vi "query 2.vi"() -> (27 "error out 2":errorcluster)   [LabVIEW 2019]
uses:
  <vilib>/Utility/NIReport.llb/Report Type.ctl
  <vilib>/addons/database/Connection.llb/DB Tools Open Connec (String).vi
  <vilib>/addons/_office/excel.llb/Excel Easy Table (str).vi
  <vilib>/addons/database/_DB Variant To Data/Database Variant To Data.xnode
  <vilib>/Utility/NIReport.llb/NI_report.lvclass
  <vilib>/addons/database/NI_Database_API.lvlib
  <vilib>/Utility/NIReport.llb/NI_ReportGenerationCore.lvlib
  <vilib>/addons/_office/NI_ReportGenerationToolkit.lvlib
  database.lvlib
panel:
  out "Table":string[][](table)
  in  "error in (no error)":errorcluster
  in  "pallet_sit sel":bool
  in  "swl sel":bool
  in  "SWR sel":bool
  in  "curv_sit sel":bool
  in  "def_type sel":bool
  in  "GB_sit sel":bool
  in  "UNTIL":timestamp
  in  "FROM":timestamp
  in  "pallet_num sel":bool
  in  "time select":bool
  in  "pallet number":i16
  in  "Pallet-sit":u16(ring) items=["normal", "warning", "error"]
  in  "CURV_SITUATION":u16(ring) items=["normal", "error"]
  in  "SWR":u16(ring) items=["normal", "error"]
  in  "SWL":u16(ring) items=["normal", "error"]
  in  "GB_SITUATION":u16(ring) items=["normal", "warning", "error"]
  in  "DEFECTS_TYPE":u16(ring) items=["gap", "hole"]
  in  "TIME":u16(ring) items=["selected period", "last day", "last week", "last mounth", "Last Turn"]
  in  "Close Square":bool
  in  "Search Button 2":bool
  in  "Save As Button 2":bool
  in  "Base Path":path=path "C:/excel files"
  # "DPIS"
  # "REPORT"
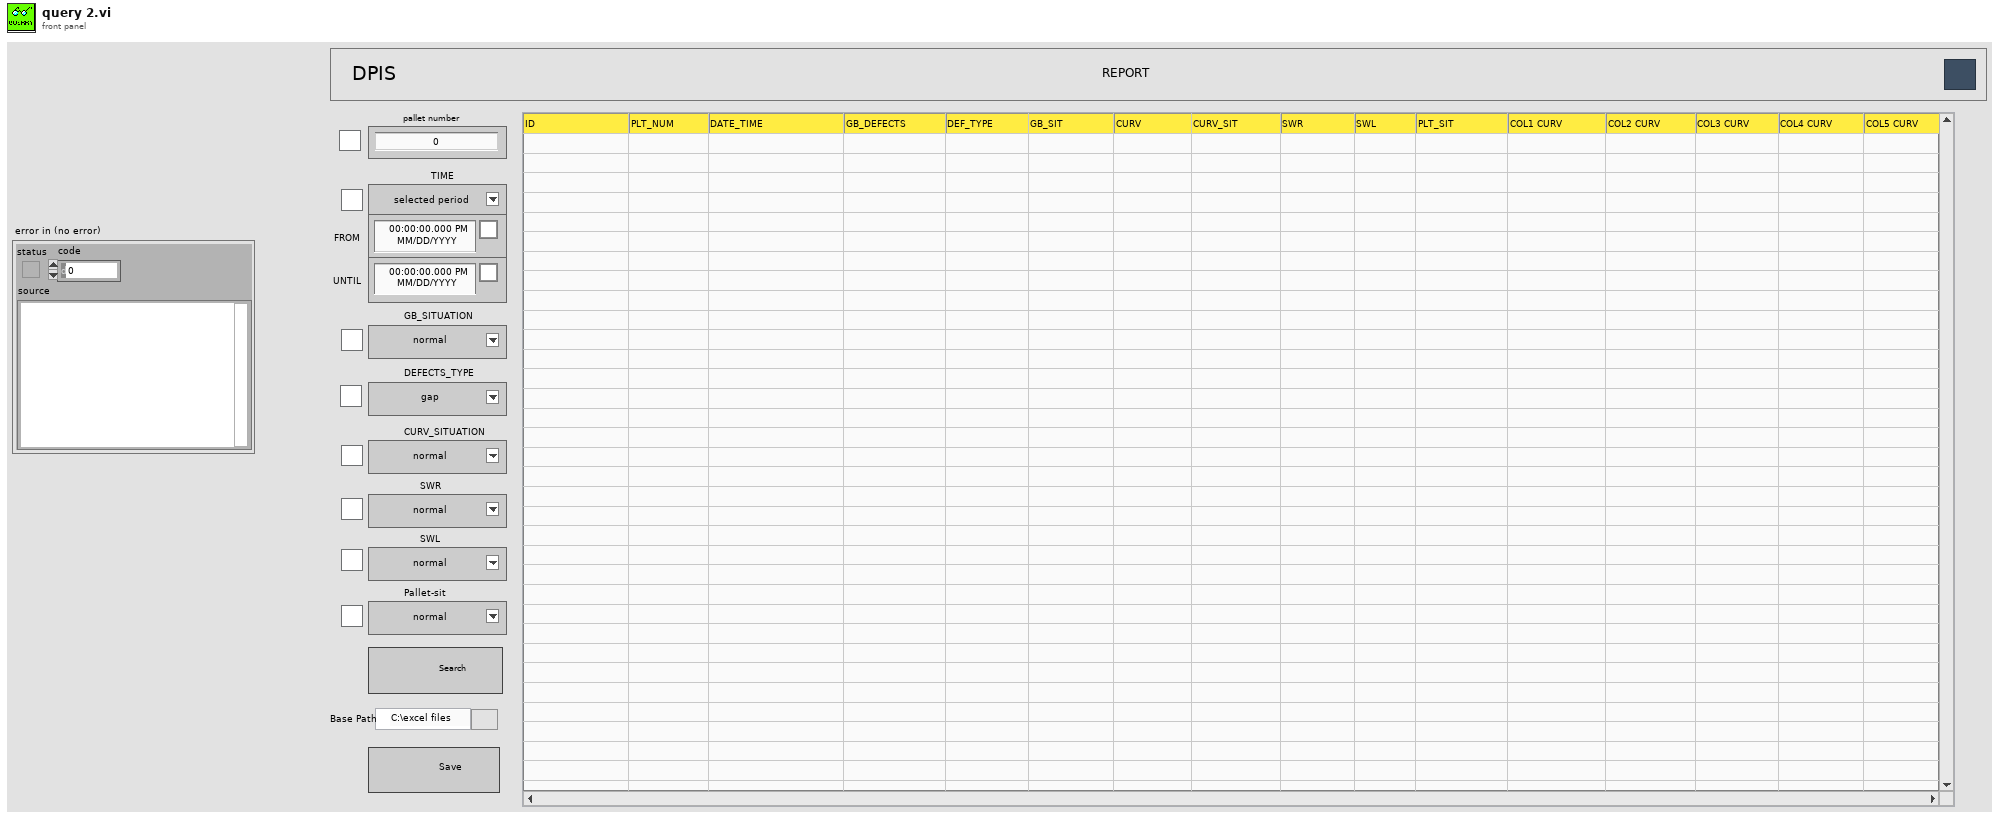
[diagram p1: front panel]
types:
  T1 = enum16{"maximized", "minimized", "normal", "no change"}
  T2 = typedef "NI_ReportGenerationCore.lvlib/Report Type.ctl" = enum16{"HTML", "Word", "Excel"}
  T3 = typedef "NI_Database_API.lvlib/Conn ObjectReference.ctl" = refnum<k1>
  T4 = cluster{"plt number dis":i16, "Table Name":string, "Database Name":string, "DB days to save":i16, "IP #":string, "Img Path":path, "Port":u16, "time out":u16, "madule path":path, "IP # speed":string, "counting device":enum16{"Sensors", "Line Speed", "Sensors&Speed"}}
  T5 = typedef "LVDateTimeRec.ctl" = cluster{"fractional second":dbl, "second":i32, "minute":i32, "hour":i32, "day of month":i32, "month":i32, "year":i32, "day of week":i32, "day of year":i32, "DST":i32}
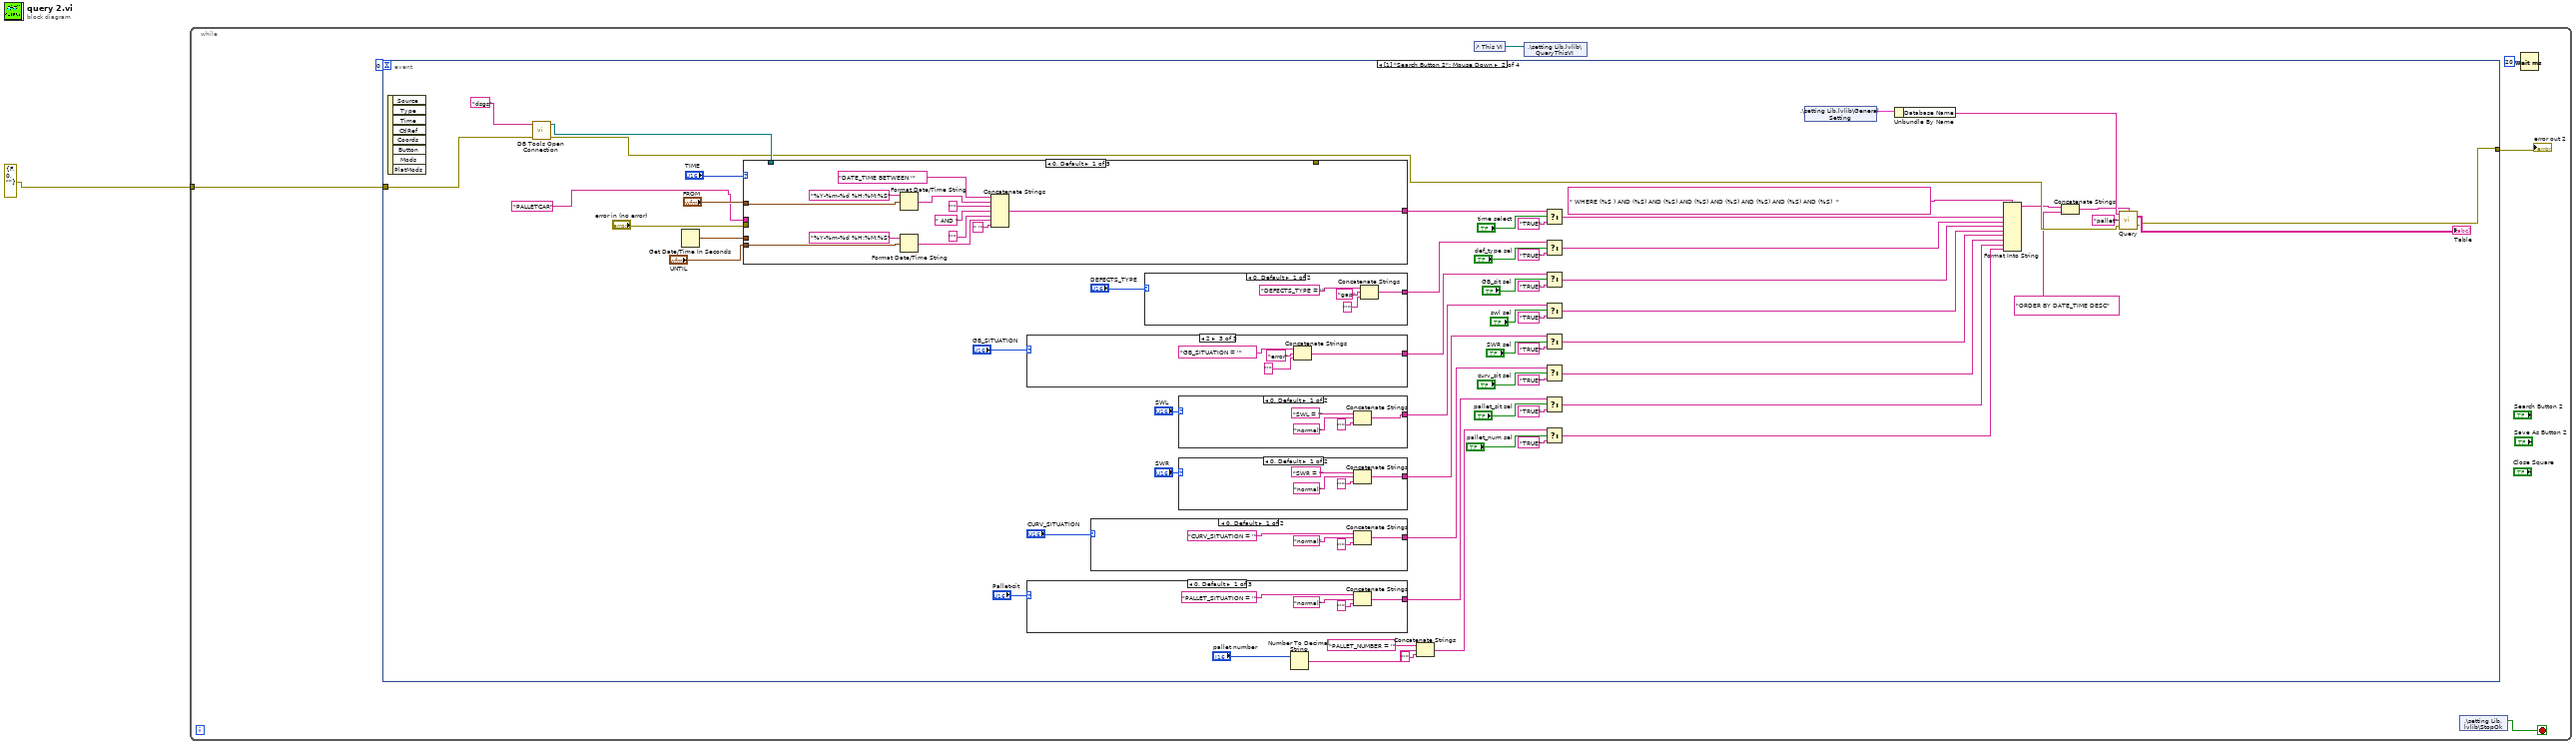
[diagram p0: block diagram]
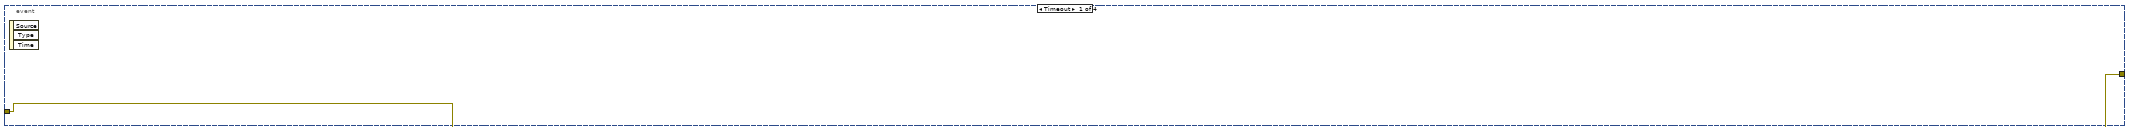
[diagram p2: hidden frame]
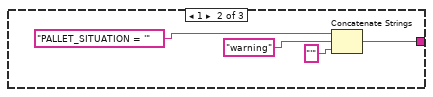
[diagram p3: hidden frame]
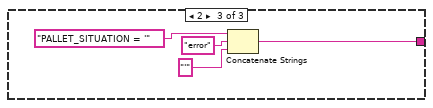
[diagram p4: hidden frame]
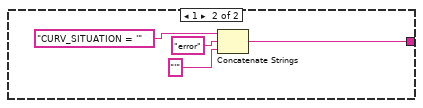
[diagram p5: hidden frame]
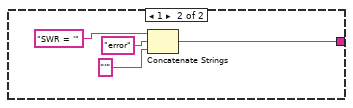
[diagram p6: hidden frame]
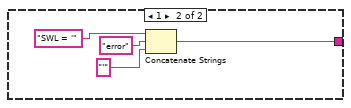
[diagram p7: hidden frame]
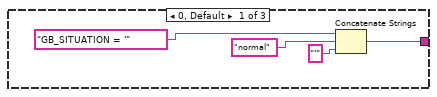
[diagram p8: hidden frame]
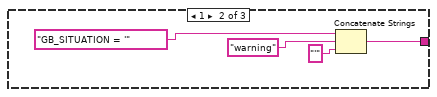
[diagram p9: hidden frame]
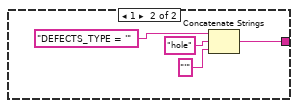
[diagram p10: hidden frame]
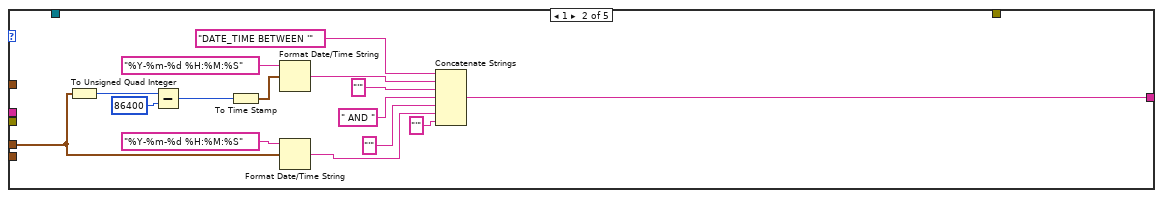
[diagram p11: hidden frame]
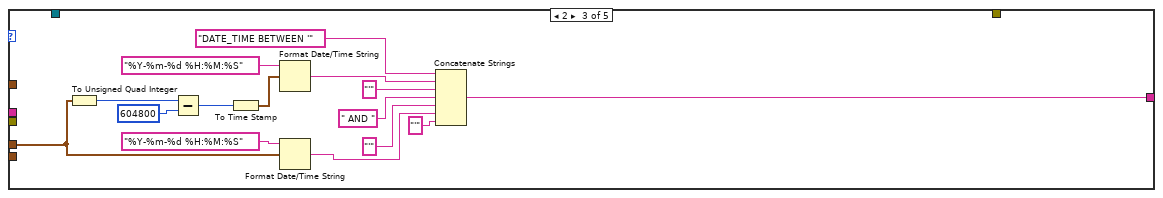
[diagram p12: hidden frame]
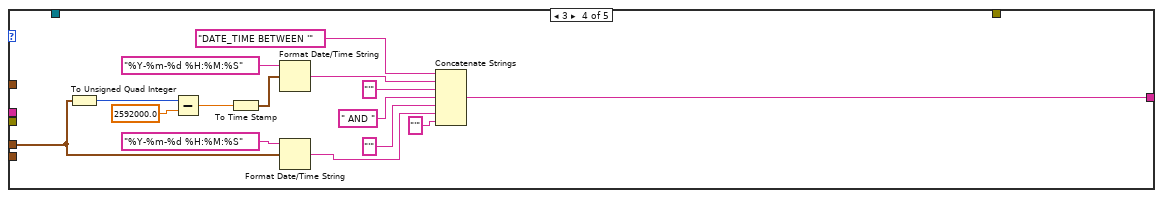
[diagram p13: hidden frame]
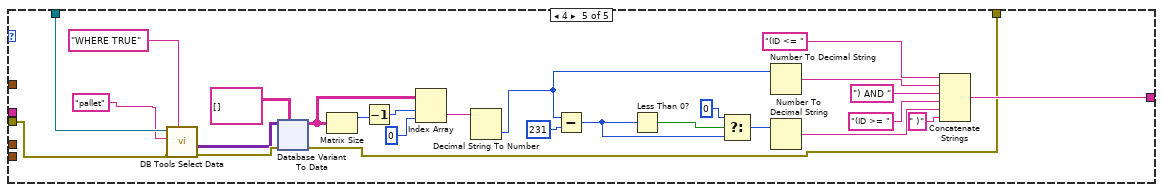
[diagram p14: hidden frame]
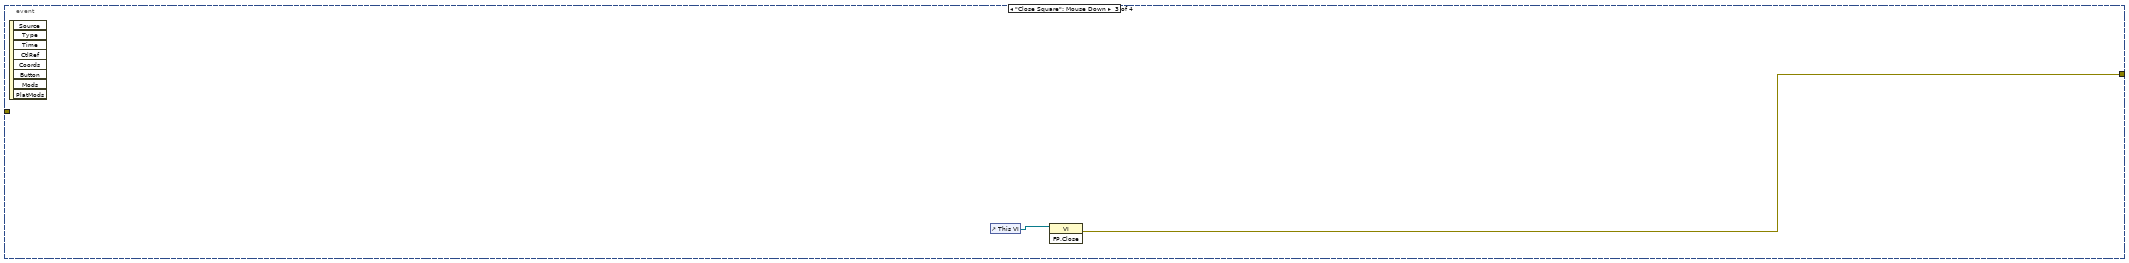
[diagram p15: hidden frame]
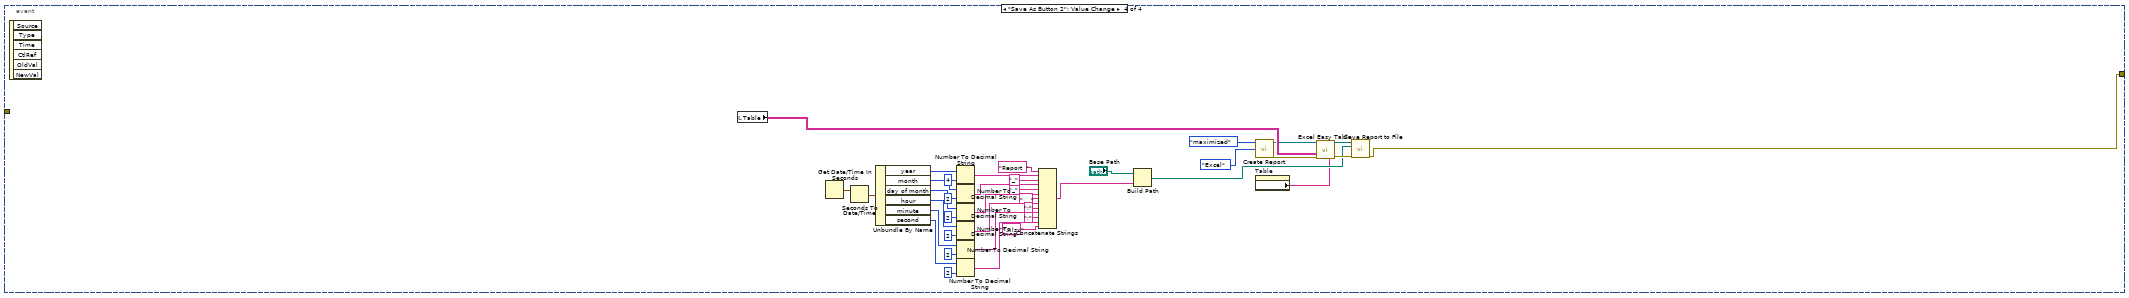
[diagram p16: hidden frame]
diagram:
  n1 = while {
    tunnel: errorcluster {"status"=FALSE, "code"=0, "source"=""} ("error in (no error)") -> [w2]
    stop <- w3 stop-if-true
    n2 = event shown="[1] \"Search Button 2\": Mouse Down" {
      selector: _ -> [_ _ _ _]
      dyn-events: _ -> [_ _ _ _]
      timeout: 0 -> [_ _ _ _]
      tunnel: [w8 w12 w253 w255] -> w4
      tunnel: w2 -> [w8 w18 _ _]
      event Timeout {
        n3 = event-data() -> ()  [unwired: 1 in, 3 out]
      }
      event "Search Button 2": Mouse Down {
        n4 = event-data() -> ()  [unwired: 1 in, 8 out]
        n5 = call-poly <vilib>:"DB Tools Open Connection.vi"("error in (no error)"=w18, "connection information"="dsgs" ("database name")) -> ("error out"=w13:errorcluster, "connection reference"=w19:T3)  [unwired: 6 in]
        n6 = Get Date/Time In Seconds() -> (seconds since 1Jan1904=w62:timestamp)
        n7 = case shown="0, Default" "TIME" {
          tunnel: "FROM" -> [w134 _ _ _ _]
          tunnel: "UNTIL" -> [w132 _ _ _ _]
          tunnel: [w127 w142 w153 w168 w193] -> w35
          tunnel: w62 -> [_ w140 w155 w170 _]
          tunnel: "error in (no error)" -> [_ _ _ _ w185]
          tunnel: [_ _ _ _ w186] -> _
          tunnel: "PALLETCAR" ("database name") -> [_ _ _ _ _]
          tunnel: w19 -> [_ _ _ _ w184]
          frame 0, Default {
            n8 = Format Date/Time String(time format string (%c)="%Y-%m-%d %H:%M:%S", seconds (now)=w134) -> (date/time string=w133:string)  [unwired: 1 in]
            n9 = Format Date/Time String(time format string (%c)="%Y-%m-%d %H:%M:%S", seconds (now)=w132) -> (date/time string=w129:string)  [unwired: 1 in]
            n10 = Concatenate Strings("DATE_TIME BETWEEN '" ("condition"), w133, "'" ("string"), " AND " ("time format string (%c)"), "'" ("string"), w129, " '" ("string")) -> (w127:string)
          }
          frame 1 {
            n11 = To Unsigned Quad Integer(1:w140) -> (0:w150:u64)
            n12 = Subtract(x=w150, y=u64 86400) -> (x-y=w152:u64)
            n13 = To Time Stamp(1:w152) -> (0:w141:timestamp)
            n14 = Format Date/Time String(time format string (%c)="%Y-%m-%d %H:%M:%S", seconds (now)=w141) -> (date/time string=w146:string)  [unwired: 1 in]
            n15 = Format Date/Time String(time format string (%c)="%Y-%m-%d %H:%M:%S", seconds (now)=w140) -> (date/time string=w143:string)  [unwired: 1 in]
            n16 = Concatenate Strings("DATE_TIME BETWEEN '" ("condition"), w146, "'" ("string"), " AND " ("time format string (%c)"), "'" ("string"), w143, "'" ("string")) -> (w142:string)
          }
          frame 2 {
            n17 = To Unsigned Quad Integer(1:w155) -> (0:w158:u64)
            n18 = Subtract(x=w158, y=u64 604800) -> (x-y=w156:u64)
            n19 = To Time Stamp(1:w156) -> (0:w154:timestamp)
            n20 = Format Date/Time String(time format string (%c)="%Y-%m-%d %H:%M:%S", seconds (now)=w154) -> (date/time string=w163:string)  [unwired: 1 in]
            n21 = Format Date/Time String(time format string (%c)="%Y-%m-%d %H:%M:%S", seconds (now)=w155) -> (date/time string=w160:string)  [unwired: 1 in]
            n22 = Concatenate Strings("DATE_TIME BETWEEN '" ("condition"), w163, "'" ("condition"), " AND " ("time format string (%c)"), "'" ("string"), w160, "'" ("string")) -> (w153:string)
          }
          frame 3 {
            n23 = To Unsigned Quad Integer(1:w170) -> (0:w172:u64)
            n24 = Subtract(x=w172, y=2592000.0) -> (x-y=w173:dbl)
            n25 = To Time Stamp(1:w173) -> (0:w169:timestamp)
            n26 = Format Date/Time String(time format string (%c)="%Y-%m-%d %H:%M:%S", seconds (now)=w169) -> (date/time string=w178:string)  [unwired: 1 in]
            n27 = Format Date/Time String(time format string (%c)="%Y-%m-%d %H:%M:%S", seconds (now)=w170) -> (date/time string=w181:string)  [unwired: 1 in]
            n28 = Concatenate Strings("DATE_TIME BETWEEN '" ("condition"), w178, "'" ("condition"), " AND " ("time format string (%c)"), "'" ("string"), w181, "'" ("string")) -> (w168:string)
          }
          frame 4 {
            n29 = call <vilib>:"DB Tools Select Data.vi"("condition"="WHERE TRUE" ("format string"), "error in (no error)"=w185, "table"="pallet", "connection reference"=w184) -> ("error out"=w208:errorcluster, "data"=w207:variant[][])  [unwired: 2 in, 1 out]
            n30 = xnode "Database Variant To Data"("database variant"=w207, "error in (no error)"=w208, "type"=string[][] []) -> ("data"=w192:string[][], "error out"=w186:errorcluster)
            n31 = Matrix Size(0:w192) -> (1:w191:i32)  [unwired: 1 out]
            n32 = Decrement(x=w191) -> (x-1=w190:i32)
            n33 = Index Array(array=w192, index (row)=w190, index (col)=0 ("disabled index (col)")) -> (element=w188:string)
            n34 = Decimal String To Number(string=w188) -> (number=w187:i32)  [unwired: 2 in, 1 out]
            n35 = Subtract(x=w187, y=231) -> (x-y=w202:i32)
            n36 = Less Than 0?(x=w202) -> (x < 0?=w201:bool)
            n37 = Select(t=0 ("y"), s=w201, f=w202) -> (s? t:f=w203:i32)
            n38 = Number To Decimal String(number=w187) -> (decimal integer string=w200:string)  [unwired: 1 in]
            n39 = Number To Decimal String(number=w203) -> (decimal integer string=w204:string)  [unwired: 1 in]
            n40 = Concatenate Strings("(ID <= " ("condition"), w200, ") AND " ("string"), "(ID >= " ("string"), w204, " )" ("string")) -> (w193:string)
          }
        }
        n41 = case shown="2" "GB_SITUATION" {
          tunnel: [w106 w110 w114] -> w49
          frame 0, Default {
            n42 = Concatenate Strings("GB_SITUATION = '" ("string"), "normal" ("string"), "'" ("string")) -> (w106:string)
          }
          frame 1 {
            n43 = Concatenate Strings("GB_SITUATION = '" ("string"), "warning" ("string"), "'" ("string")) -> (w110:string)
          }
          frame 2 {
            n44 = Concatenate Strings("GB_SITUATION = '" ("string"), "error" ("string"), "'" ("string")) -> (w114:string)
          }
        }
        n45 = case shown="0, Default" "Pallet-sit" {
          tunnel: [w70 w74 w78] -> w41
          frame 0, Default {
            n46 = Concatenate Strings("PALLET_SITUATION = '" ("string"), "normal" ("string"), "'" ("string")) -> (w70:string)
          }
          frame 1 {
            n47 = Concatenate Strings("PALLET_SITUATION = '" ("string"), "warning" ("string"), "'" ("string")) -> (w74:string)
          }
          frame 2 {
            n48 = Concatenate Strings("PALLET_SITUATION = '" ("string"), "error" ("string"), "'" ("string")) -> (w78:string)
          }
        }
        n49 = case shown="0, Default" "CURV_SITUATION" {
          tunnel: [w82 w86] -> w43
          frame 0, Default {
            n50 = Concatenate Strings("CURV_SITUATION = '" ("string"), "normal" ("string"), "'" ("string")) -> (w82:string)
          }
          frame 1 {
            n51 = Concatenate Strings("CURV_SITUATION = '" ("string"), "error" ("string"), "'" ("string")) -> (w86:string)
          }
        }
        n52 = case shown="0, Default" "DEFECTS_TYPE" {
          tunnel: [w118 w122] -> w56
          frame 0, Default {
            n53 = Concatenate Strings("DEFECTS_TYPE = '" ("string"), "gap" ("string"), "'" ("string")) -> (w118:string)
          }
          frame 1 {
            n54 = Concatenate Strings("DEFECTS_TYPE = '" ("string"), "hole" ("string"), "'" ("string")) -> (w122:string)
          }
        }
        n55 = case shown="0, Default" "SWL" {
          tunnel: [w98 w102] -> w47
          frame 0, Default {
            n56 = Concatenate Strings("SWL = '" ("string"), "normal" ("string"), "'" ("string")) -> (w98:string)
          }
          frame 1 {
            n57 = Concatenate Strings("SWL = '" ("string"), "error" ("string"), "'" ("string")) -> (w102:string)
          }
        }
        n58 = case shown="0, Default" "SWR" {
          tunnel: [w90 w94] -> w45
          frame 0, Default {
            n59 = Concatenate Strings("SWR = '" ("string"), "normal" ("string"), "'" ("string")) -> (w90:string)
          }
          frame 1 {
            n60 = Concatenate Strings("SWR = '" ("string"), "error" ("string"), "'" ("string")) -> (w94:string)
          }
        }
        n61 = Number To Decimal String(number="pallet number") -> (decimal integer string=w61:string)  [unwired: 1 in]
        n62 = Concatenate Strings("PALLET_NUMBER = '" ("string"), w61, "'" ("string")) -> (w39:string)
        n63 = Select(t=w35, s="time select", f="TRUE") -> (s? t:f=w34:string)
        n64 = Select(t=w56, s="def_type sel", f="TRUE") -> (s? t:f=w33:string)
        n65 = Select(t=w49, s="GB_sit sel", f="TRUE") -> (s? t:f=w32:string)
        n66 = Select(t=w47, s="swl sel", f="TRUE") -> (s? t:f=w31:string)
        n67 = Select(t=w45, s="SWR sel", f="TRUE") -> (s? t:f=w30:string)
        n68 = Select(t=w43, s="curv_sit sel", f="TRUE") -> (s? t:f=w29:string)
        n69 = Select(t=w41, s="pallet_sit sel", f="TRUE") -> (s? t:f=w28:string)
        n70 = Select(t=w39, s="pallet_num sel", f="TRUE") -> (s? t:f=w27:string)
        n71 = shared-variable ".\\setting Lib.lvlib\\General Setting"() -> (w17:T4)  [unwired: 1 in, 1 out]
        n72 = Unbundle By Name(w17) -> ("Database Name"=w16:string)
        n73 = Format Into String(format string=" WHERE (%S ) AND (%S) AND (%S) AND (%S) AND (%S) AND (%S) AND (%S) AND (%S)  ", w34, w33, w32, w31, w30, w29, w28, w27) -> (resulting string=w11:string)  [unwired: 2 in, 1 out]
        n74 = Concatenate Strings(w11, "ORDER BY DATE_TIME DESC" ("string")) -> (w9:string)
        n75 = call "Query.vi"("Condition"=w9, "Error in"=w13, "Table Name"="pallet", "Connection Name"=w16) -> ("Error out"=w12:errorcluster, "data"=→"Table":string[][])
      }
      event "Close Square": Mouse Down {
        n76 = event-data() -> ()  [unwired: 1 in, 8 out]
        n77 = control-ref of="This VI"() -> (w254:refnum<vi>)
        n78 = invoke class="VI" method="FP.Close"(reference=w254) -> (error out=w253:errorcluster)  [unwired: 2 in, 2 out]
      }
      event "Save As Button 2": Value Change {
        n79 = event-data() -> ()  [unwired: 1 in, 6 out]
        n80 = local read "Table"() -> (w293:string[][])
        n81 = Get Date/Time In Seconds() -> (seconds since 1Jan1904=w290:timestamp)
        n82 = Seconds To Date/Time(time stamp (now)=w290) -> (date time rec=w289:T5)  [unwired: 1 in]
        n83 = Unbundle By Name(w289) -> ("year"=w288:i32, "month"=w287:i32, "day of month"=w286:i32, "hour"=w285:i32, "minute"=w284:i32, "second"=w283:i32)
        n84 = Number To Decimal String(number=w288, width (-)=i16 4) -> (decimal integer string=w282:string)
        n85 = Number To Decimal String(number=w287, width (-)=i16 2) -> (decimal integer string=w280:string)
        n86 = Number To Decimal String(number=w286, width (-)=i16 2) -> (decimal integer string=w278:string)
        n87 = Number To Decimal String(number=w285, width (-)=i16 2) -> (decimal integer string=w276:string)
        n88 = Number To Decimal String(number=w284, width (-)=i16 2) -> (decimal integer string=w274:string)
        n89 = Number To Decimal String(number=w283, width (-)=i16 2) -> (decimal integer string=w272:string)
        n90 = Concatenate Strings("Report  " ("string"), w282, "_" ("string"), w280, "_" ("string"), w278, "    " ("string"), w276, ";" ("string"), w274, ";" ("string"), w272, ".xlsx" ("string")) -> (w270:string)
        n91 = Build Path(base path="Base Path", name or relative path=w270) -> (appended path=w260:path)
        n92 = property on="Table" class="Tbl (strict)"() -> ("Column Headers[]"=w257:string[])  [unwired: 2 in, 2 out]
        n93 = call <vilib>:"Create Report.vi"("window state (normal)"=T1."maximized", "report type"=Report_Type."Excel") -> ("report out"=w259:refnum<class "NI_report.lvclass">, "error out"=w258:errorcluster)  [unwired: 12 in]
        n94 = call-poly <vilib>:"Excel Easy Table.vi"("report in"=w259, "text data"=w293, "error in (no error)"=w258, "column headers"=w257) -> ("report out"=w261:refnum<class "NI_report.lvclass">, "error out"=w262:errorcluster)  [unwired: 7 in, 3 out]
        n95 = call-dynamic "Save Report to File.vi"("report in"=w261, "report file path"=w260, "error in (no error)"=w262) -> ("error out"=w255:errorcluster)  [unwired: 11 in, 1 out]
      }
    }
    "error out 2" <- w4
    n96 = control-ref of="This VI"() -> (w5:refnum<vi>)
    n97 = shared-variable ".\\setting Lib.lvlib\\QueryThisVI"(w5) -> ()  [unwired: 1 in, 1 out]
    n98 = shared-variable ".\\setting Lib.lvlib\\StopOk"() -> (w3:bool)  [unwired: 1 in, 1 out]
    n99 = Wait (ms)(milliseconds to wait=u32 20) -> ()  [unwired: 1 out]
  }
